vi "Exit.vi"(8 "error in":errorcluster) -> (0 "error out":errorcluster)   [LabVIEW 2018, in "GUI.lvclass"]
uses:
  GUI.lvclass
  Queue/Queue Data.ctl
  Queue/State.ctl
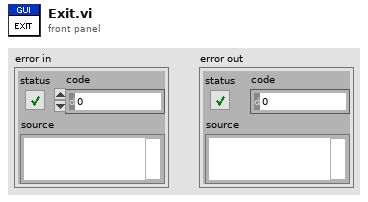
[diagram p1: front panel]
types:
  T1 = typedef "GUI.lvclass/Queue Data.ctl" = cluster{"State":T2, "Data":variant}
  T2 = typedef "GUI.lvclass/State.ctl" = enum16{"Initialize", "LoadConfig", "SaveConfig", "S1Alarm", "S2Alarm", "S1EndOfTest", "S2EndOfTest", "Monitor", "Error", "Exit"}
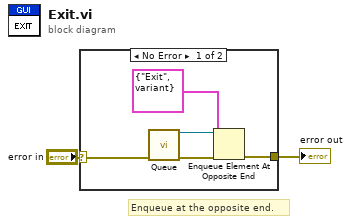
[diagram p0: block diagram]
diagram:
  # "Enqueue at the opposite end."
  n1 = case shown="No Error" "error in" {
    selector: "error in" -> [w7 w8]
    tunnel: [w4 w8] -> w2
    frame No Error {
      n2 = call "Queue.vi"("error in"=w7) -> ("error out"=w6:errorcluster, "queue out"=w5:refnum<queue>)  [unwired: 9 in]
      n3 = Enqueue Element At Opposite End(queue=w5, element=T1 {"State"=enum."Exit", "Data"=variant}, error in (no error)=w6) -> (error out=w4:errorcluster)  [unwired: 1 in, 2 out]
    }
    frame Error {
    }
  }
  "error out" <- w2
